vi "Receive - UDP (SAP).vi"() -> ()   [LabVIEW 2020]
uses:
  <instrlib>/AIM GmbH/_AIM 664/_controls/comm_verification_rx.ctl
  <instrlib>/AIM GmbH/_AIM 664/_controls/sap_config_rx.ctl
  <instrlib>/AIM GmbH/_AIM 664/_polimorphicInstances/session/CreateSession(Rx-VL-Oriented).vi
  <instrlib>/AIM GmbH/_AIM 664/bsp/AFDX_Receive/Create Rx VL.vi
  <instrlib>/AIM GmbH/_AIM 664/_polimorphicInstances/udpPort/CreateUdpPort(RX-SAP).vi
  <instrlib>/AIM GmbH/_AIM 664/_polimorphicInstances/control/Start (Rx).vi
  <instrlib>/AIM GmbH/_AIM 664/_polimorphicInstances/control/Stop (Rx).vi
  <instrlib>/AIM GmbH/_AIM 664/_polimorphicInstances/session/CleanupSession (Port).vi
  <instrlib>/AIM GmbH/_AIM 664/AIM664LV.lvlib
panel:
  in  "Period mS":u32=200
  out "MsgRead":u32
  out "Data":u8[](array[numeric])=[1, 2, 3, 4, 0, 0, 0, 0, 0, 0, 0, 0, 0, 0, 0, 0, 0, 0, 0, 0, 0, 0, 0, 0, 0, 0, 0, 0, 0, 0, 0, 0, 0, 0, 0, 0, 0, 0, 0, 0, 0, 0, 0, 0, 0, 0, 0, 0, 0, 0, 0, 0, 0, 0, 0, 0, 0, 0, 0, 0, 0, 0, 0, 0, 0, 0, 0, 0, 0, 0, 0, 0, 0, 0, 0, 0, 0, 0, 0, 0, 0, 0, 0, 0, 0, 0, 0, 0, 0, 0, 0, 0, 0, 0, 0, 0, 0, 0, 0, 0] format="%.0x"
  in  "Messages to Read (1)":u32=1
  in  "SapPort Config":T1={"UdpDstPort"=12345, "UdpNumBufMessages"=0, "UdpMaxMessageSize"=0}
  in  "VL Config":T2={"VlId"=0, "VLRange"=0, "VerificationMode"=0, "Bag"=0, "Jitter"=0, "MaxFrameLength"=0, "MaxSkew"=0, "VLBufSize"=32768, "FilterMode"=0, "FilterPosition"=0, "Padding"=0, "FilterMask"=0, "FilterData"=0, "MinFrameLength"=0} {"FilterMode" items=["FDX_RX_VL_FLT_DIS", "FDX_RX_VL_FLT_ENA ", "FDX_RX_VL_FLT_ENA_INV"]; "VerificationMode" items=["FDX_RX_VL_CHECK_ENA_DEFAULT"=65535, "FDX_RX_VL_CHECK_REDMAM"=16, "DX_RX_VL_CHECK_TRAFIC"=8, "FDX_RX_VL_CHECK_FRAMESIZE"=4, "FDX_RX_VL_CHECK_SNINTEG"=2, "FDX_RX_VL_CHECK_INVPAC"=1, "FDX_RX_VL_CHECK_DISA"=0]}
  out "PortInitOut":T3 {"PortConfig" items=["FDX_SINGLE", "FDX_REDUNDANT"]}
  in  "port":u32
  in  "board":u32
  out "error out":errorcluster
  in  "stop":bool
  out "current time":timestamp
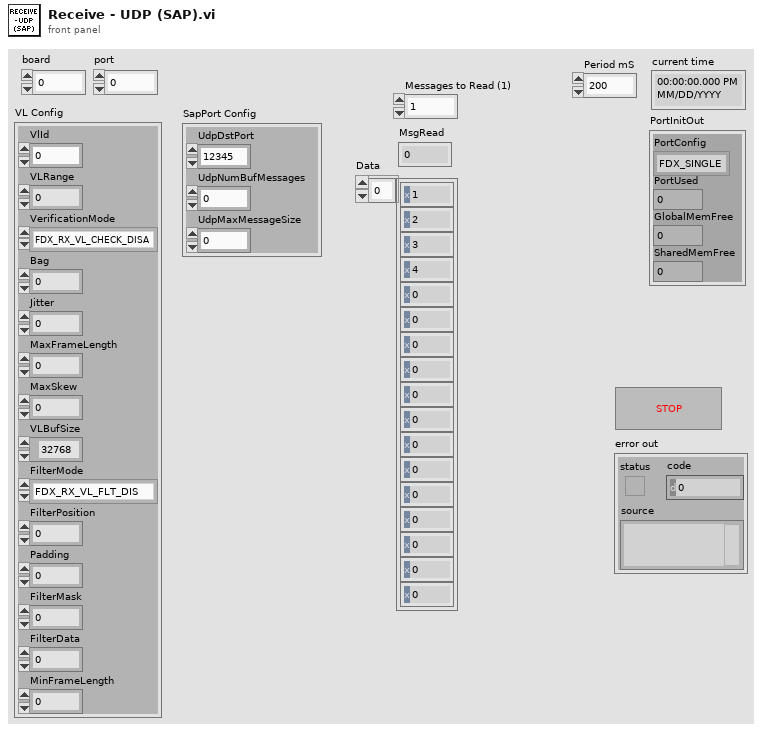
[diagram p1: front panel]
types:
  T1 = typedef "AIM664LV.lvlib/sap_config_rx.ctl" = cluster{"UdpDstPort":u16, "UdpNumBufMessages":u32, "UdpMaxMessageSize":u32}
  T2 = typedef "AIM664LV.lvlib/comm_verification_rx.ctl" = cluster{"VlId":u16, "VLRange":u32, "VerificationMode":u32, "Bag":u32, "Jitter":u32, "MaxFrameLength":u32, "MaxSkew":u32, "VLBufSize":u32, "FilterMode":u32, "FilterPosition":u32, "Padding":u32, "FilterMask":u32, "FilterData":u32, "MinFrameLength":u32}
  T3 = cluster{"PortConfig":u32, "PortUsed":u32, "GlobalMemFree":u32, "SharedMemFree":u32}
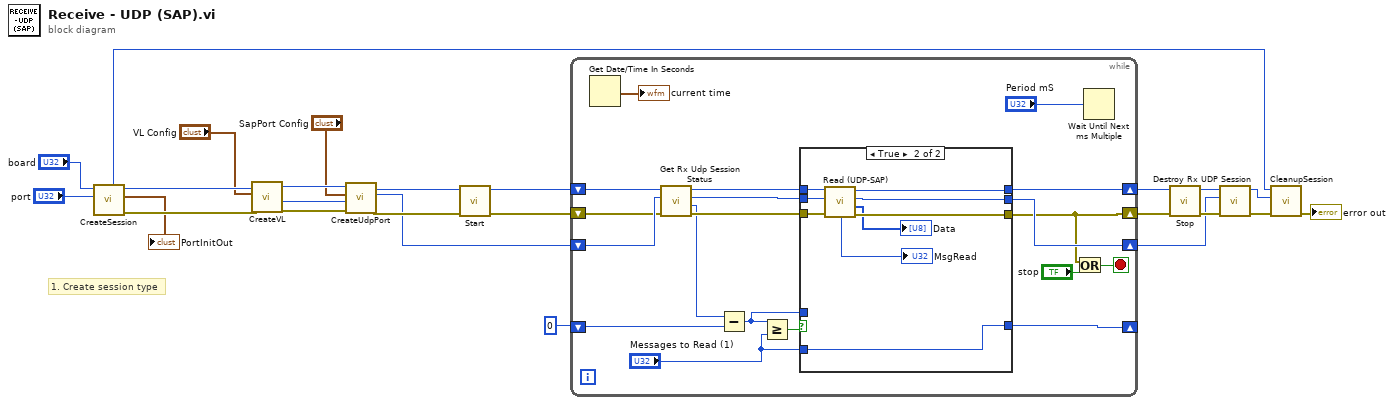
[diagram p0: block diagram]
diagram:
  # "1. Create session type"
  n1 = call-poly <instrlib>:"CreateSession.vi"("port"="port", "board"="board") -> ("error out"=w24:errorcluster, "PortInitOut"=→"PortInitOut":T3, "InstrumentHandle_port out"=w25:u32, "InstrumentHandle_board out"=w3:u32)  [unwired: 4 in, 2 out]
  n2 = call-poly <instrlib>:"CreateVL.vi"("error in (no error)"=w24, "VL Config"="VL Config", "InstrumentHandle_port in"=w25) -> ("error out"=w22:errorcluster, "VlId"=w7:u16, "InstrumentHandle_port out"=w23:u32)  [unwired: 6 in]
  n3 = call-poly <instrlib>:"CreateUdpPort.vi"("error in (no error)"=w22, "VlId"=w7, "SapPort Config"="SapPort Config", "port handle in"=w23) -> ("error out"=w20:errorcluster, "sapPort handle out"=w17:u32, "port handle out"=w21:u32)  [unwired: 4 in, 1 out]
  n4 = call-poly <instrlib>:"Start.vi"("error in (no error)"=w20, "InstrumentHandle_port in"=w21) -> ("error out"=w2:errorcluster, "InstrumentHandle_port out"=w19:u32)  [unwired: 8 in]
  n5 = while {
    shift-right: [w34] -> w18
    shift-left: w19 -> [w35]
    shift-right: [w31] -> w6
    shift-left: w17 -> [w33]
    shift-right: [w37] -> _
    shift-left: u32 0 ("MsgCount") -> [w43]
    shift-right: [w27] -> w1
    shift-left: w2 -> [w30]
    stop <- w26 stop-if-true
    n6 = Get Date/Time In Seconds() -> (seconds since 1Jan1904=→"current time":timestamp)
    n7 = call <instrlib>:"Get Rx Udp Session Status.vi"("error in (no error)"=w30, "UdpHandle in"=w33, "InstrumentHandle_port in"=w35) -> ("error out"=w42:errorcluster, "MsgCount"=w36:u32, "UdpHandle out"=w32:u32, "InstrumentHandle_port out"=w41:u32)  [unwired: 4 in, 1 out]
    n8 = Subtract(x=w36, y=w43) -> (x-y=w38:u32)
    n9 = Greater Or Equal?(x=w38, y="Messages to Read (1)") -> (x >= y?=w40:bool)
    n10 = case shown="True" w40 {
      tunnel: w42 -> [w46 w55]
      tunnel: w41 -> [w48 w56]
      tunnel: "Messages to Read (1)" -> [_ w57]
      tunnel: [w48 w54] -> w34
      tunnel: w38 -> [w47 _]
      tunnel: [w47 w57] -> w37
      tunnel: [w46 w53] -> w27
      tunnel: w32 -> [w45 w52]
      tunnel: [w45 w51] -> w31
      frame False {
      }
      frame True {
        n11 = call <instrlib>:"Read (UDP-SAP).vi"("error in"=w55, "UdpHandle in"=w52, "InstrumentHandle_port in"=w56) -> ("error out"=w53:errorcluster, "Data"=→"Data":u8[], "UdpHandle out"=w51:u32, "InstrumentHandle_port out"=w54:u32, "MsgRead"=→"MsgRead":u32)  [unwired: 4 in]
      }
    }
    n12 = Or(x=w27, y="stop") -> (x .or. y?=w26:bool)
    n13 = Wait Until Next ms Multiple(millisecond multiple="Period mS") -> ()  [unwired: 1 out]
  }
  n14 = call-poly <instrlib>:"Stop.vi"("error in (no error)"=w1, "InstrumentHandle_port in"=w18) -> ("error out"=w16:errorcluster, "InstrumentHandle_port out"=w5:u32)  [unwired: 8 in]
  n15 = call <instrlib>:"Destroy Rx UDP Session.vi"("error in (no error)"=w16, "UdpHandle in"=w6, "InstrumentHandle_port in"=w5) -> ("error out"=w15:errorcluster, "InstrumentHandle_port out"=w4:u32)  [unwired: 7 in]
  n16 = call-poly <instrlib>:"CleanupSession.vi"("error in (no error)"=w15, "InstrumentHandle_port in"=w4, "InstrumentHandle_board in"=w3) -> ("error out"=→"error out":errorcluster)  [unwired: 8 in]
